vi "本地控制.vi"() -> (2 "远程2":bool)   [LabVIEW 2015]
panel:
  in  "远程":bool
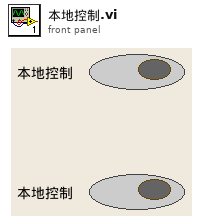
[diagram p1: front panel]
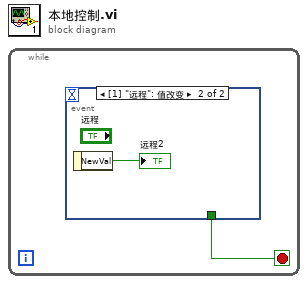
[diagram p0: block diagram]
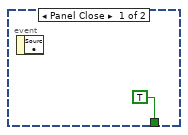
[diagram p2: hidden frame]
diagram:
  n1 = while {
    stop <- w1 stop-if-true
    n2 = event shown="[1] \"远程\": 值改变" {
      selector: _ -> [_ _]
      dyn-events: _ -> [_ _]
      timeout: _ -> [_ _]
      tunnel: [TRUE _] -> w1
      event Panel Close {
        n3 = event-data() -> ()  [unwired: 1 in, 1 out]
      }
      event "远程": Value Change {
        n4 = event-data() -> ("NewVal"=→"远程2":bool)  [unwired: 1 in]
      }
    }
  }
